vi "configure write to Spartan INI.vi"(8 "error in (no error)":errorcluster, 9 "Value (\"\")":string, 10 "Key (\"\")":string, 11 "Section (\"Spartan Server\")":string="Spartan Server") -> (0 "error out":errorcluster)   [LabVIEW 2011]
uses:
  <vilib>/Utility/config.llb/Write Key (String).vi
  <vilib>/Utility/config.llb/NI_LVConfig.lvlib
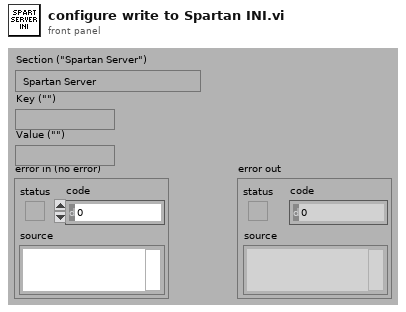
[diagram p1: front panel]
types:
  T1 = typedef "NI_LVConfig.lvlib/Config Data RefNum.ctl" = refnum<k1>
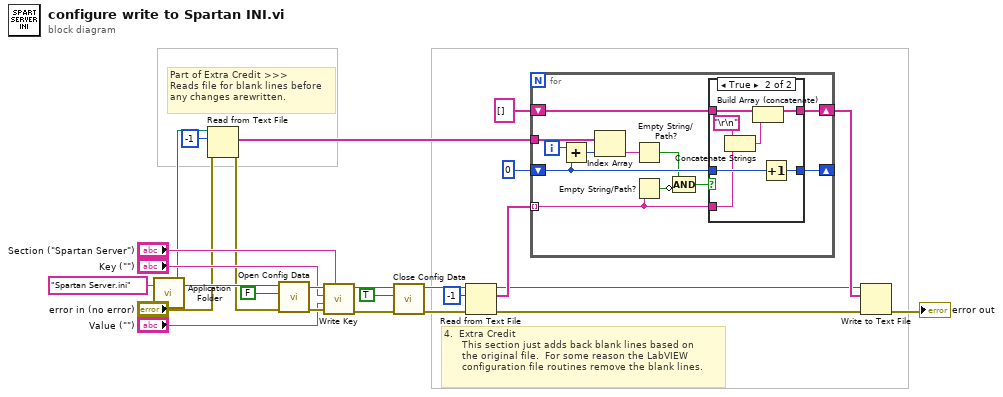
[diagram p0: block diagram]
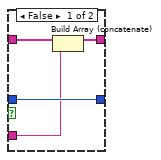
[diagram p2: hidden frame]
diagram:
  # "Part of Extra Credit >>>\nReads file for blank lines before\nany changes arewritten."
  # "4.  Extra Credit\n      This section just adds back blank lines based on\n      the original file.  For some reason the LabVIEW\n      configuration file routines remove the blank lines."
  n1 = call "Application Folder.vi"("Relative Path (\"\" - Folder)"="Spartan Server.ini" ("section")) -> ("Application Folder"=w5:path)  [unwired: 2 in]
  n2 = Read from Text File(file (use dialog)=w5, count=-1, error in="error in (no error)") -> (text=w1:string[], error out=w3:errorcluster)  [unwired: 1 in, 2 out]
  n3 = call <vilib>:"Open Config Data.vi"("error in (no error)"=w3, "create file if necessary (T)"=FALSE ("create file if necessary? (T)"), "configuration file path"=w5) -> ("error out"=w23:errorcluster, "refnum"=w24:T1)  [unwired: 6 in, 1 out]
  n4 = call-poly <vilib>:"Write Key.vi"("section"="Section (\"Spartan Server\")", "error in (no error)"=w23, "value"="Value (\"\")", "key"="Key (\"\")", "refnum"=w24) -> ("error out"=w21:errorcluster, "refnum out"=w22:T1)  [unwired: 1 in, 4 out]
  n5 = call <vilib>:"Close Config Data.vi"("error in (no error)"=w21, "write file if changed (T)"=TRUE ("write configuration file? (T)"), "refnum"=w22) -> ("error out"=w7:errorcluster, "file path"=w2:path)  [unwired: 7 out]
  n6 = Read from Text File(file (use dialog)=w2, count=-1, error in=w7) -> (text=w8:string[], error out=w12:errorcluster)  [unwired: 1 in, 2 out]
  n7 = for {
    tunnel: w1 -> [w33]
    shift-right: [w35] -> w9
    shift-left: string[] [] -> [w36]
    shift-right: [w34] -> _
    shift-left: 0 -> [w30]
    tunnel: w8 -> [w27] mode=indexing
    i -> [w31]
    n8 = Add(x=w31, y=w30) -> (x+y=w29:i32)
    n9 = Index Array(array=w33, index=w29) -> (element=w32:string)
    n10 = Empty String/Path?(string/path=w32) -> (empty?=w26:bool)
    n11 = Empty String/Path?(string/path=w27) -> (empty?=w28:bool)
    n12 = Compound Arithmetic op=AND(w26, invert w28) -> (w25:bool)
    n13 = case shown="True" w25 {
      tunnel: w36 -> [w40 w47]
      tunnel: [w39 w46] -> w35
      tunnel: w30 -> [w38 w45]
      tunnel: [w38 w44] -> w34
      tunnel: w27 -> [w37 w42]
      frame False {
        n14 = Build Array (concatenate)(w40, w37) -> (w39:string[])
      }
      frame True {
        n15 = Concatenate Strings("\r\n", w42) -> (w41:string)
        n16 = Build Array (concatenate)(w47, w41) -> (w46:string[])
        n17 = Increment(x=w45) -> (x+1=w44:i32)
      }
    }
  }
  n18 = Write to Text File(file (use dialog)=w2, text=w9, error in=w12) -> (error out=→"error out":errorcluster)  [unwired: 1 in, 2 out]
